vi "JoySticks.vi"   [LabVIEW 2019]
uses:
  <vilib>/Rock Robotics/WPI/Joystick/WPI_JoystickDeviceEnum.ctl
  Globals/JoyStick Global.vi
types:
  T1 = typedef "WPI_JoystickDeviceEnum.ctl" = enum16{"USB 0", "USB 1", "USB 2", "USB 3", "USB 4", "USB 5"}
  T2 = typedef "WPI_JoystickDevRef.ctl" = cluster{"Device":T1}
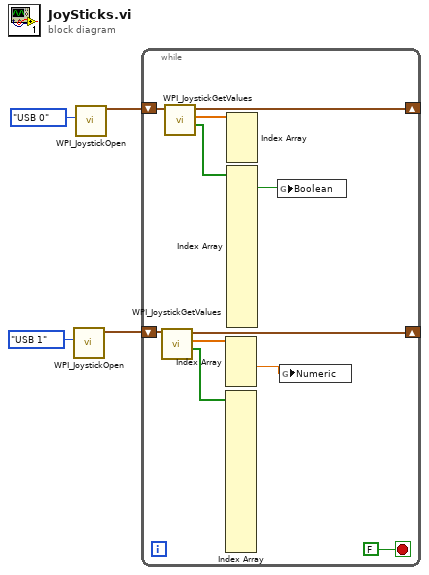
[diagram p0: block diagram]
diagram:
  n1 = call <vilib>:"WPI_JoystickOpen.vi"("JoystickDevice"=WPI_JoystickDeviceEnum."USB 1") -> ("JoystickDevRef"=w1:T2)  [unwired: 10 in]
  n2 = call <vilib>:"WPI_JoystickOpen.vi"("JoystickDevice"=WPI_JoystickDeviceEnum."USB 0") -> ("JoystickDevRef"=w2:T2)  [unwired: 10 in]
  n3 = while {
    shift-right: [w15] -> _
    shift-left: w2 -> [w14]
    shift-right: [w12] -> _
    shift-left: w1 -> [w13]
    stop <- FALSE stop-if-true
    n4 = call <vilib>:"WPI_JoystickGetValues.vi"("JoystickDevRef"=w13) -> ("Buttons"=w8:bool[], "Axes"=w9:dbl[], "JoystickDevRef"=w12:T2)  [unwired: 6 in, 2 out]
    n5 = call <vilib>:"WPI_JoystickGetValues.vi"("JoystickDevRef"=w14) -> ("Buttons"=w10:bool[], "Axes"=w11:dbl[], "JoystickDevRef"=w15:T2)  [unwired: 6 in, 2 out]
    n6 = Index Array(array=w9) -> (element #2=w5:dbl)  [unwired: 4 in, 3 out]
    n7 = Index Array(array=w8) -> ()  [unwired: 18 in, 18 out]
    n8 = Index Array(array=w11) -> ()  [unwired: 4 in, 4 out]
    n9 = Index Array(array=w10) -> (element #1=w7:bool)  [unwired: 18 in, 17 out]
    n10 = global write "JoyStick Global.vi" "Boolean"(w7) -> ()
    n11 = global write "JoyStick Global.vi" "Numeric"(w5) -> ()
  }
